vi "Configure Comparator Tolerance.vi"(5 "BIN High Limit (0.0)":dbl, 7 "BIN Low Limit (0.0)":dbl, 8 "error in (no error)":errorcluster, 9 "BIN No. (0:None)":u16(ring) items=["None", "BIN1", "BIN2", "BIN3", "BIN4", "BIN5", "BIN6", "BIN7", "BIN8", "BIN9"], 10 "Nominal Value (0.0)":dbl, 11 "VISA resource name":refnum<visa-resource-name>) -> (0 "error out":errorcluster, 3 "VISA resource name out":refnum<visa-resource-name>)   [LabVIEW 2017, in "Agilent E4980.lvlib"]
doc: "Sets the nominal value, low limit and high limit values for the comparator operation.\n\n<B>Notes:</B>\n(1) This is valid only when you select the limit mode as tolerance."
uses:
  Agilent E4980.lvlib
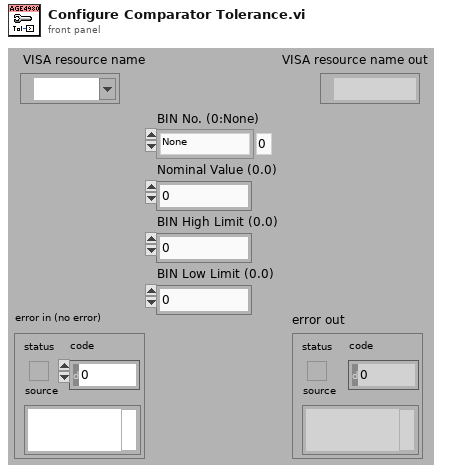
[diagram p1: front panel]
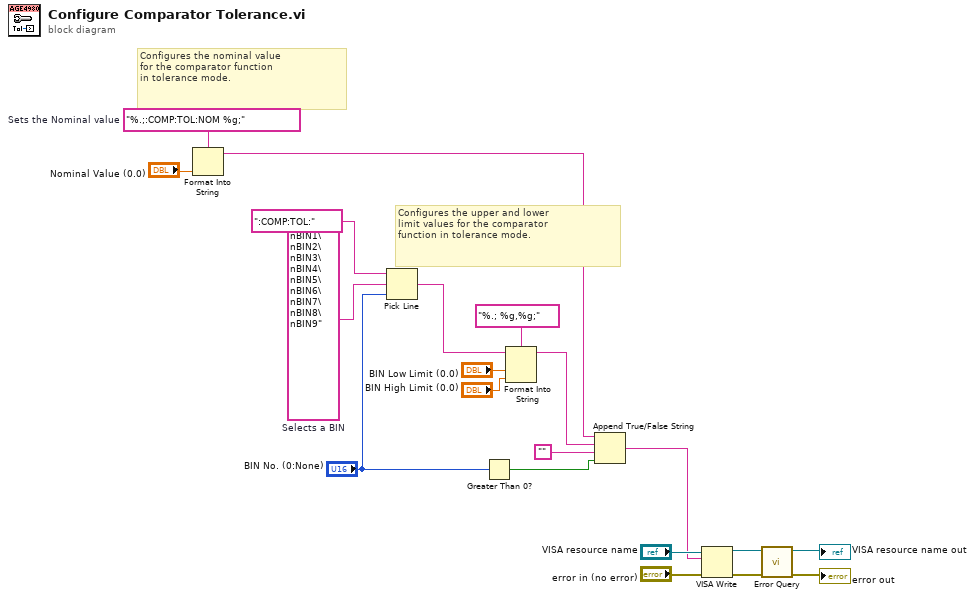
[diagram p0: block diagram]
diagram:
  w16 = "NONE\nBIN1\nBIN2\nBIN3\nBIN4\nBIN5\nBIN6\nBIN7\nBIN8\nBIN9"  # Selects a BIN
  w19 = "%.;:COMP:TOL:NOM %g;"  # Sets the Nominal value
  # "Configures the upper and lower\nlimit values for the comparator\nfunction in tolerance mode."
  # "Configures the nominal value\nfor the comparator function\nin tolerance mode."
  n1 = Format Into String(format string=w19, "Nominal Value (0.0)") -> (resulting string=w2:string)  [unwired: 2 in, 1 out]
  n2 = Pick Line(string ("")=":COMP:TOL:", multi-line string=w16, line index="BIN No. (0:None)") -> (output string=w15:string)
  n3 = Greater Than 0?(x="BIN No. (0:None)") -> (x > 0?=w9:bool)
  n4 = Format Into String(format string="%.; %g,%g;", initial string=w15, "BIN Low Limit (0.0)", "BIN High Limit (0.0)") -> (resulting string=w11:string)  [unwired: 1 in, 1 out]
  n5 = Append True/False String(1:w9, 2:"" ("Empty String Constant"), 3:w11, 4:w2) -> (0:w1:string)
  n6 = VISA Write(VISA resource name="VISA resource name", write buffer=w1, error in (no error)="error in (no error)") -> (VISA resource name out=w6:refnum<visa-resource-name>, error out=w5:errorcluster)  [unwired: 1 out]
  n7 = call "Error Query.vi"("error in (no error)"=w5, "VISA resource name"=w6) -> ("error out"=→"error out":errorcluster, "VISA resource name out"=→"VISA resource name out":refnum<visa-resource-name>)  [unwired: 6 in, 2 out]
